vi "S7NetCom Simple Test Harness.vi"() -> ()   [LabVIEW 2014]
doc: "____\nCopyright (c) 2019 Hampel Software Engineering (HSE), released under BSD license. More info can be found on https://dokuwiki.hampel-soft.com/code/hse/s7netcom. Original code published by Marc Christenson, Sisu Devices."
uses:
  Controls/S7_Variable_Type.ctl
  Controls/S7_Memory_Area.ctl
  Controls/S7_Start_Address.ctl
  API/Write Data - Boolean (Scalar).vi
  API/Write Data - String.vi
  API/Write Data - DTL (Scalar).vi
  API/Write Data - Siemens Date & Time (Scalar).vi
  API/Write Data - Byte (Scalar).vi
  API/Write Data - Word (Scalar).vi
  API/Write Data - Real (Scalar).vi
  API/Write Data - Real (1D Array).vi
  API/Read Data - Boolean (Scalar).vi
  API/Read Data - String.vi
  API/Read Data - DTL (Scalar).vi
  API/Read Data - Siemens Date&Time (Scalar).vi
  API/Read Data - Byte (Scalar).vi
  API/Read Data - Word (Scalar).vi
  API/Read Data - Real (Scalar).vi
  API/Read Data - Real (1D Array).vi
  S7NetCom.lvclass
panel:
  in  "Cont TO":i32=250
  in  "Count":u16=1 caption="Read Length"
  out "Seq No":u16
  in  "RAW Var Type":T1=enum."BYTE"
  in  "Memory Area":T2=132 items=["P Area"=128, "I Area"=129, "O Area"=130, "M Area"=131, "DB Area"=132, "Counter"=40, "Timer"=41]
  in  "Start Address":T3
  in  "Data Block #":u16=1
  in  "Bit Offset":u8
  in  "Cont Variable Type":T1=enum."BYTE" caption="Variable Type"
  in  "Cont Memory Area":T2=132 caption="Memory Area" items=["P Area"=128, "I Area"=129, "O Area"=130, "M Area"=131, "DB Area"=132, "Counter"=40, "Timer"=41]
  in  "Cont Start Address":T3 caption="Start Address"
  in  "Cont Read Length":u16=1 caption="Read Length"
  in  "Cont Data Block #":u16=1 caption="Data Block #"
  in  "Cont Bit Offset":u8 caption="Bit Offset"
  in  "Tab Control TX":T4(tab)
  in  "TX Data":u32[](array[numeric])
  in  "Btn_WriteRaw":bool
  in  "Btn_WriteBOOL":bool
  in  "Boolean Value (TX)":bool
  out "Boolean Value (RX)":bool
  in  "Btn_ReadBOOL":bool
  in  "Btn_WriteBYTE":bool
  in  "Byte Value (TX)":u8
  out "Byte Value (RX)":u8
  in  "Btn_ReadBYTE":bool
  in  "Btn_WriteWORD":bool
  in  "Word Value (TX)":u16
  out "Word Value (RX)":u16
  in  "Btn_ReadWORD":bool
  in  "Btn_WriteREAL":bool
  in  "Real Value (TX)":sgl
  out "Real Value (RX)":sgl
  in  "Btn_ReadREAL":bool
  in  "Real Values (TX)":sgl[](array[numeric])
  in  "Btn_WriteREALArray":bool
  in  "Btn_ReadREALArray":bool
  out "Real Values (RX)":sgl[](array[numeric])
  in  "String Read Length":u16
  out "String Value (RX)":string
  in  "String Value (TX)":string
  in  "Btn_WriteSTRING":bool
  in  "Btn_ReadSTRING":bool
  in  "Btn_ReadDTL":bool
  out "DTL Value (RX)":timestamp
  in  "DTL (TX)":timestamp
  in  "Btn_Write DTL":bool
  in  "Date & Time (TX)":timestamp
  in  "Btn_Write D&T":bool
  in  "Btn_ReadD&T":bool
  out "Date&Time Value (RX)":timestamp
  out "Read/Write Error out":errorcluster
  out "Real (32bit)":sgl
  in  "Rack":u8
  out "Bits (1st byte)":bool[](array[boolean])
  out "Char's":string[](array[string])
  out "String":string
  in  "stop":bool
  out "U32":i32[](array[numeric]) format="%.0x"
  out "Error out":errorcluster caption="Read Continuously Error out"
  in  "IP Address":string
  in  "Port":i32=102
  in  "Slot":u8
  in  "Timeout":i32=5000
  # "Connection"
  # "Read Continuously"
  # "Read / Write"
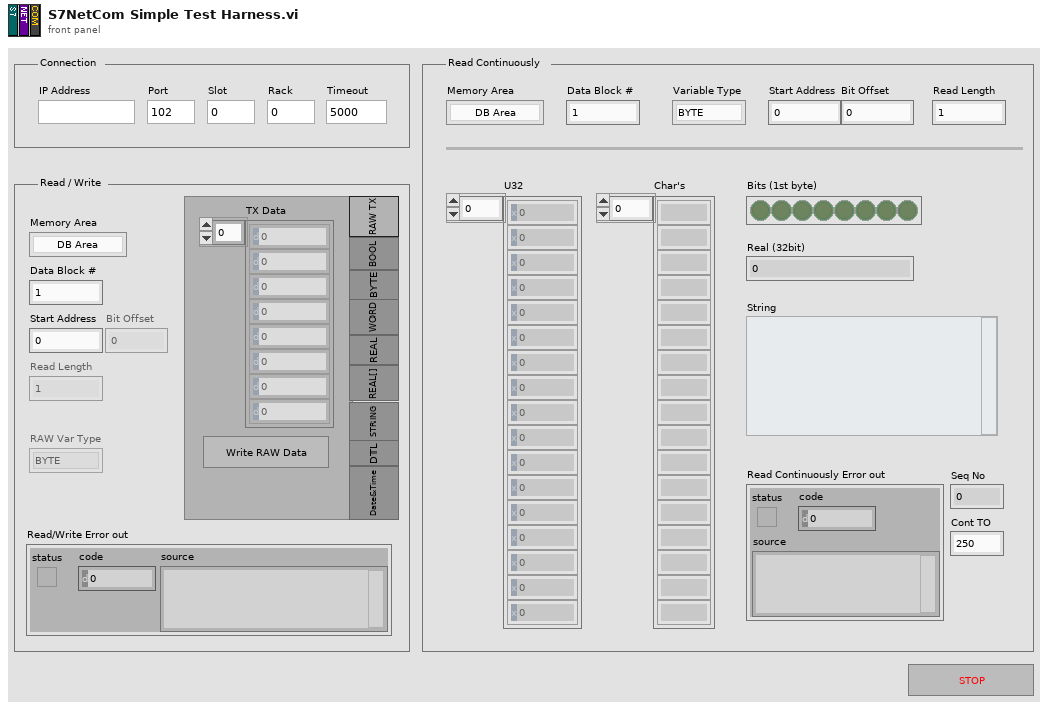
[diagram p1: front panel]
types:
  T1 = typedef "S7NetCom.lvclass/S7_Variable_Type.ctl" = enum8{"---", "BIT", "BYTE", "CHAR", "WORD", "INT", "DWORD", "DINT", "REAL"}
  T2 = typedef "S7NetCom.lvclass/S7_Memory_Area.ctl" = u8
  T3 = typedef "S7NetCom.lvclass/S7_Start_Address.ctl" = u16
  T4 = enum32{"RAW TX", "BOOL", "BYTE", "WORD", "REAL", "REAL[]", "STRING", "DTL", "Date&Time"}
  T5 = enum8{"Enabled", "Disabled", "Disabled and Grayed Out"}
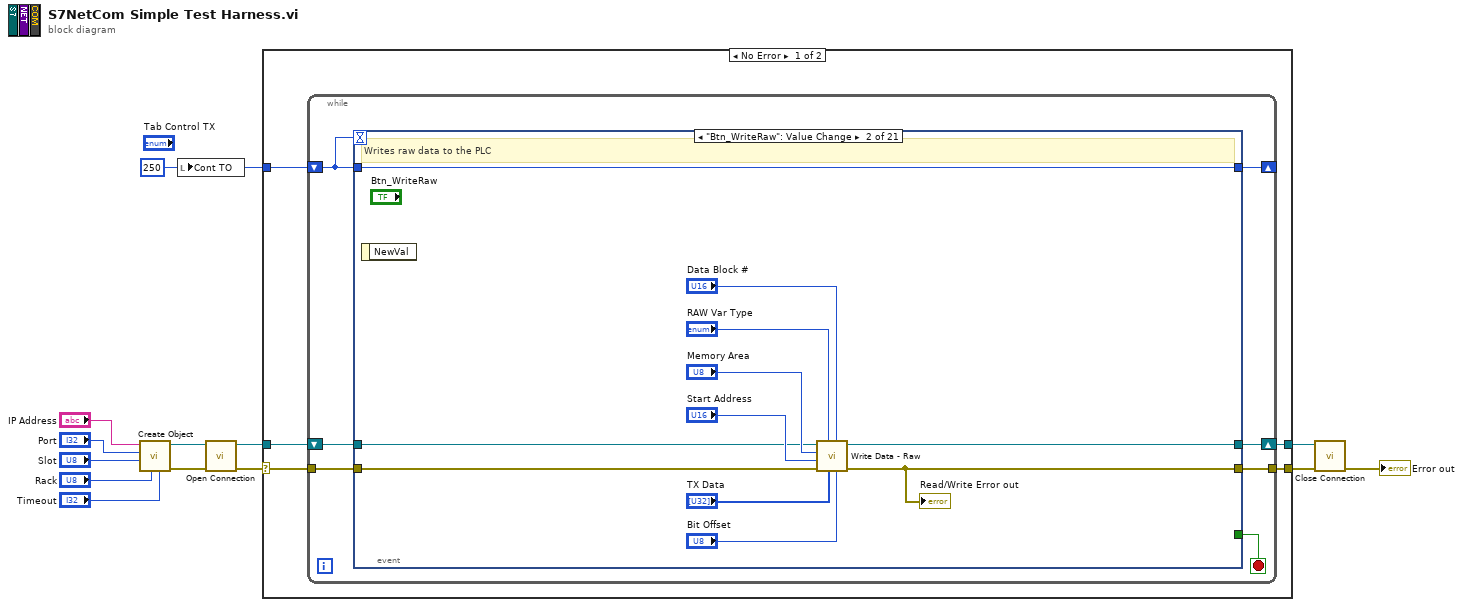
[diagram p0: block diagram]
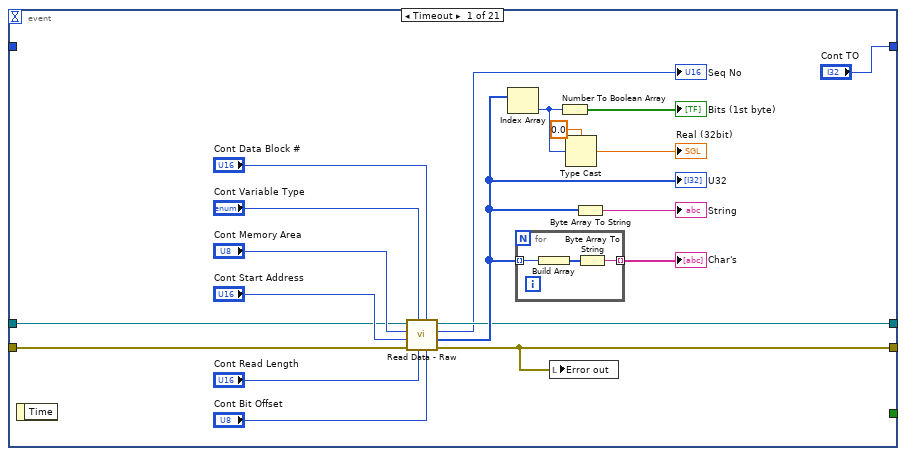
[diagram p2: hidden frame]
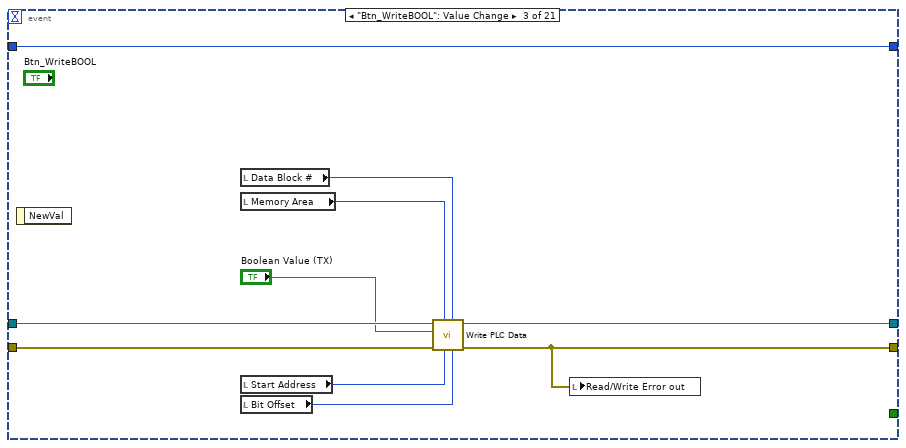
[diagram p3: hidden frame]
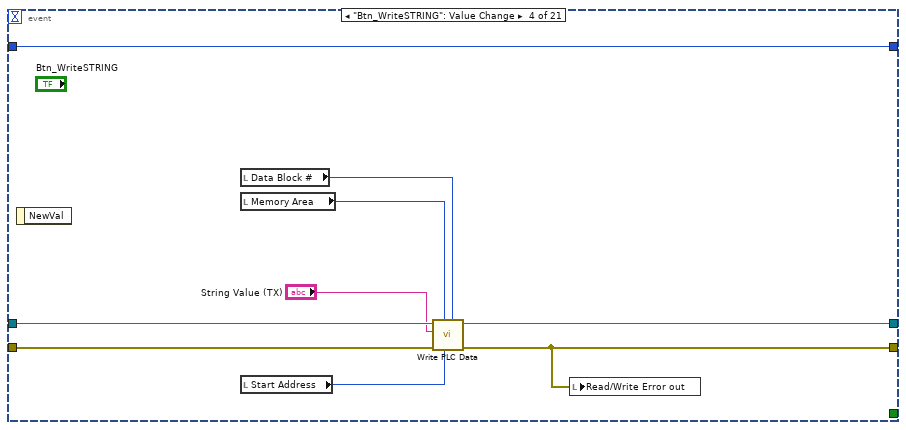
[diagram p4: hidden frame]
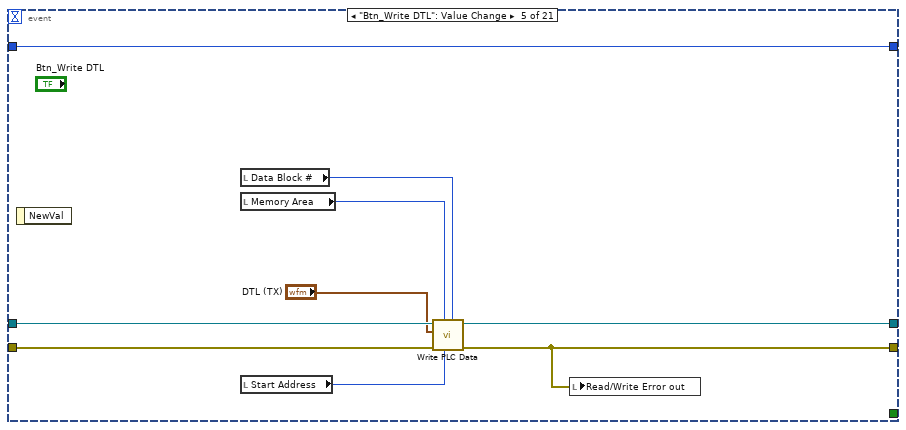
[diagram p5: hidden frame]
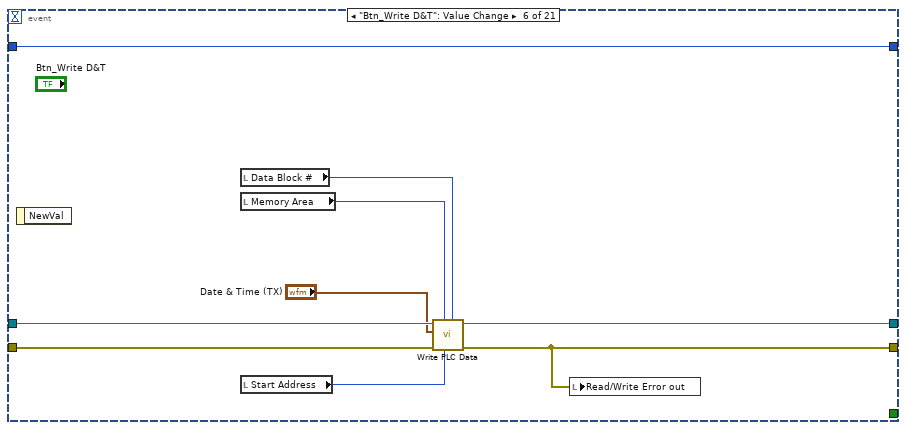
[diagram p6: hidden frame]
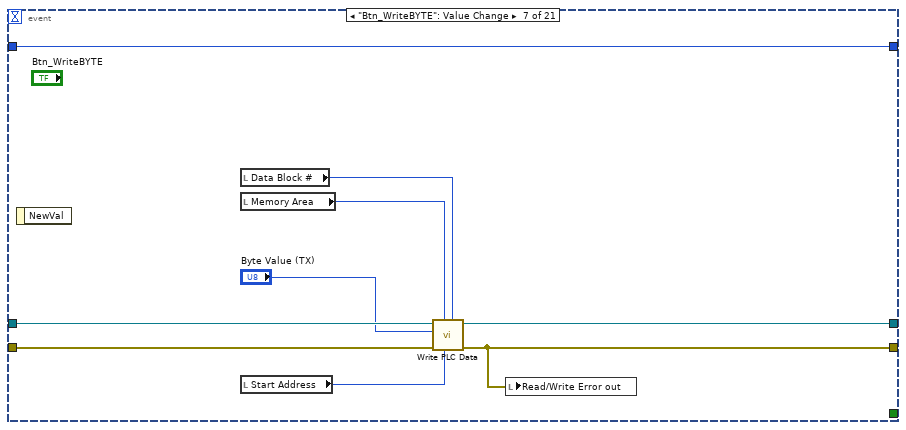
[diagram p7: hidden frame]
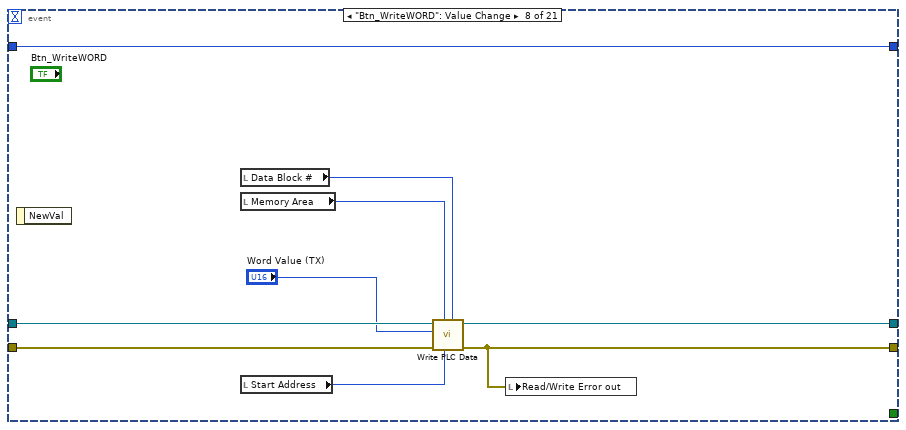
[diagram p8: hidden frame]
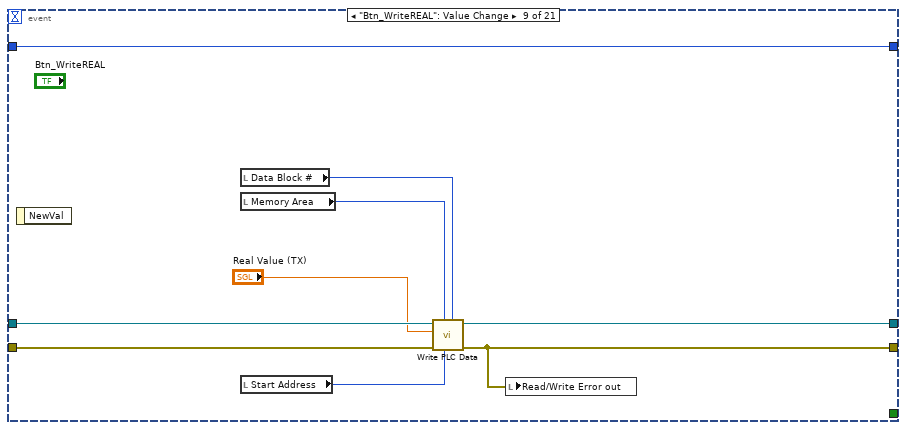
[diagram p9: hidden frame]
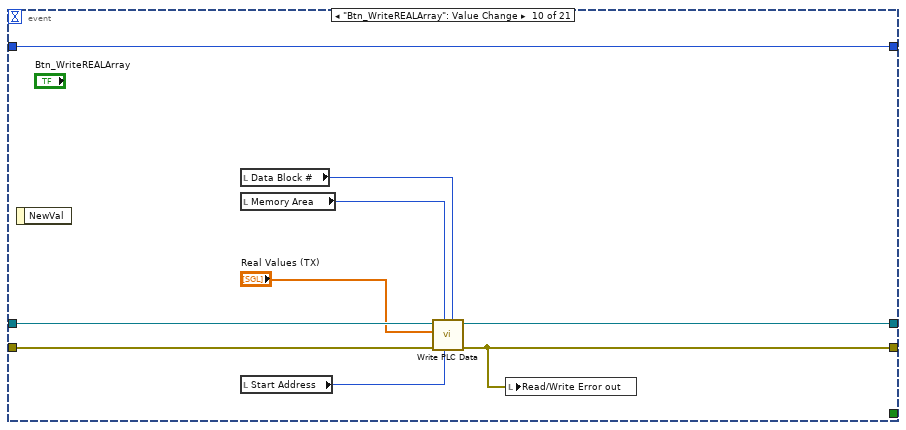
[diagram p10: hidden frame]
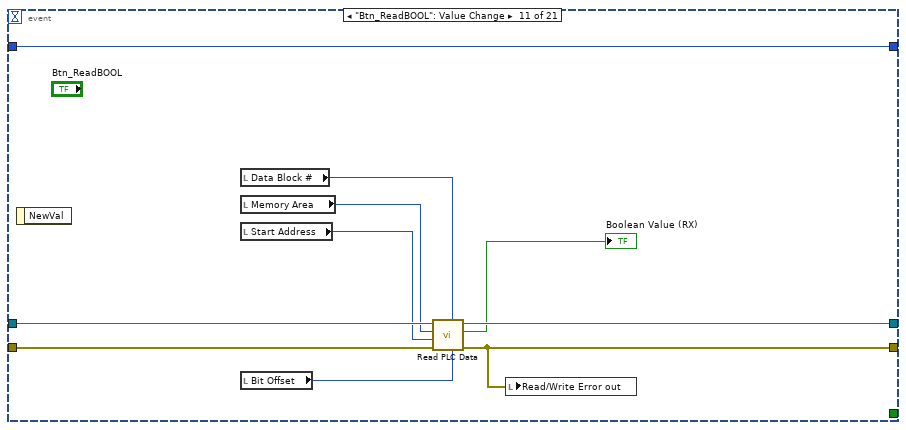
[diagram p11: hidden frame]
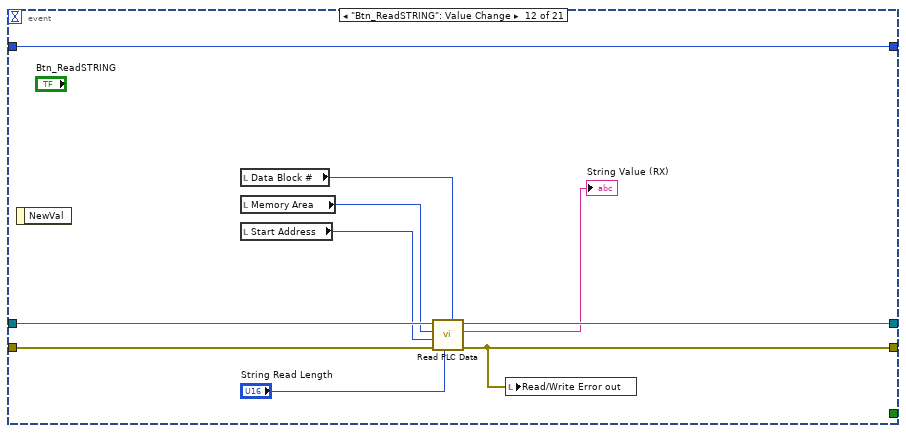
[diagram p12: hidden frame]
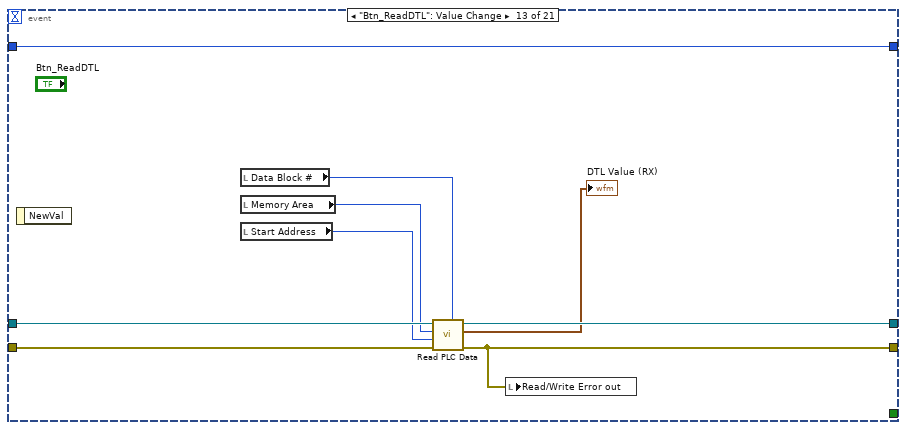
[diagram p13: hidden frame]
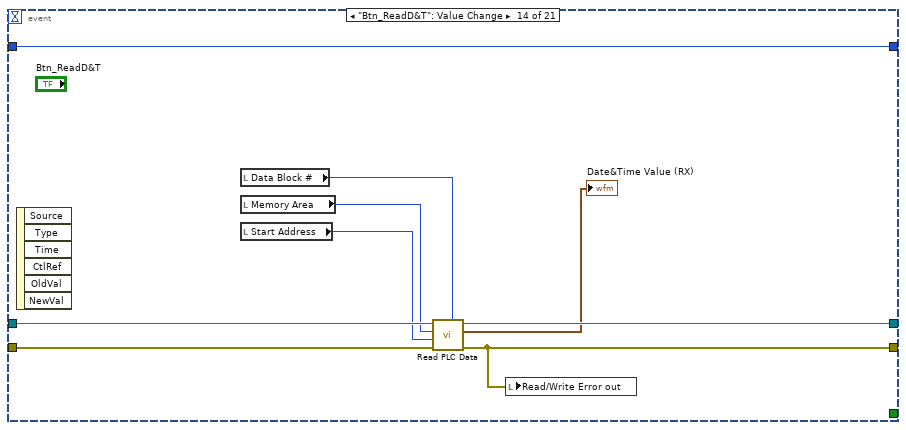
[diagram p14: hidden frame]
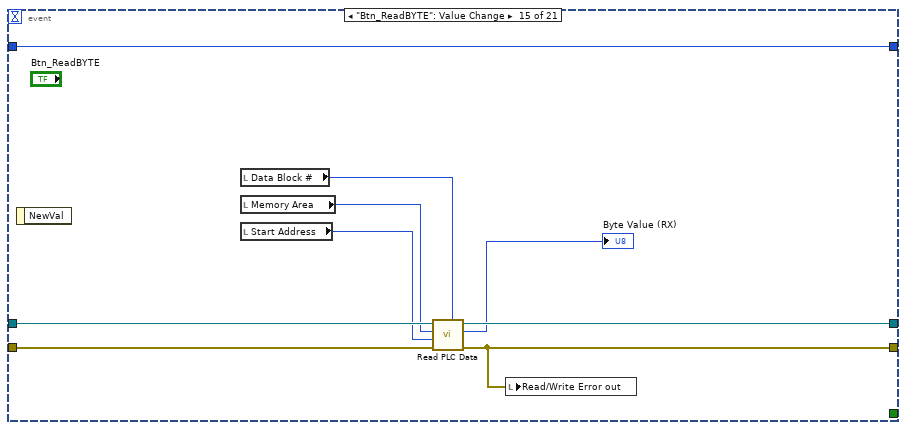
[diagram p15: hidden frame]
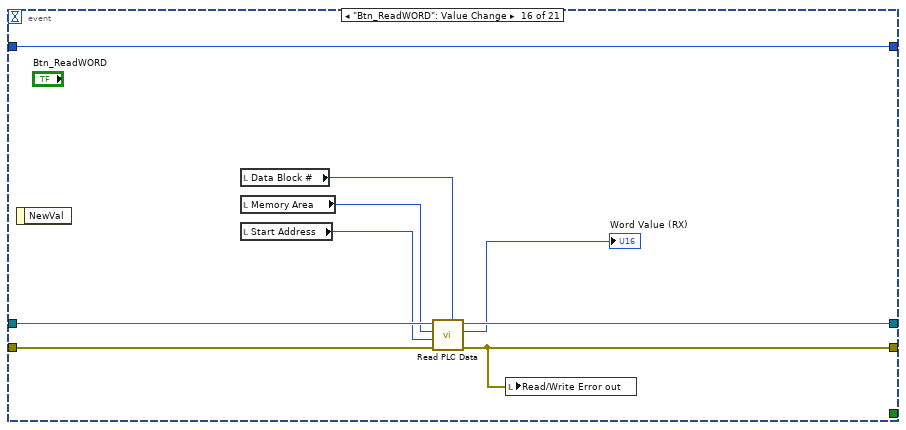
[diagram p16: hidden frame]
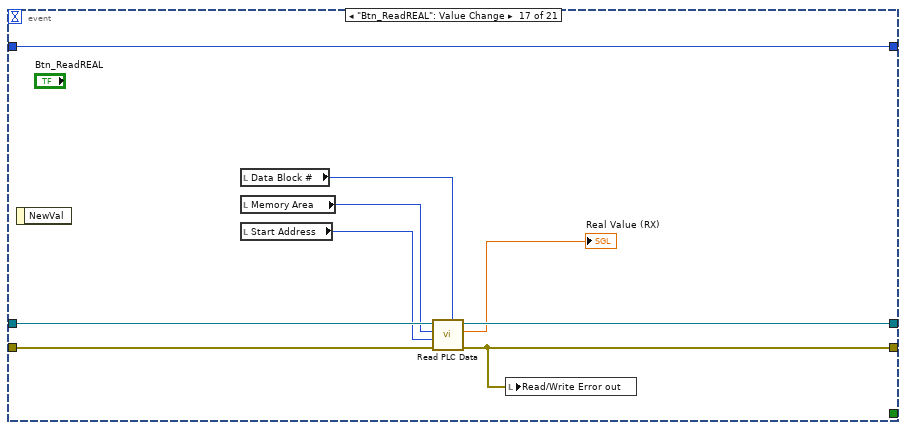
[diagram p17: hidden frame]
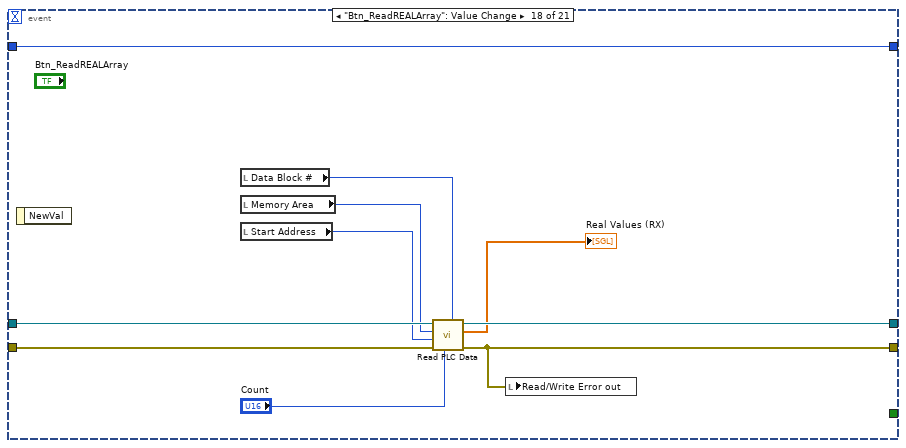
[diagram p18: hidden frame]
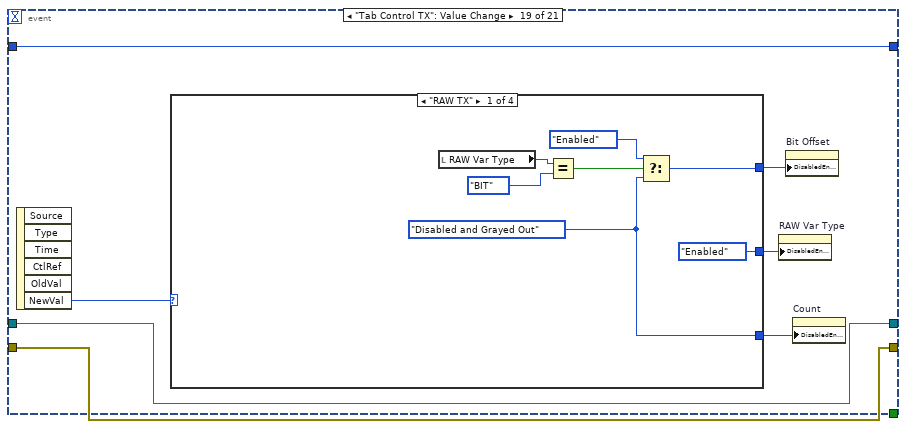
[diagram p19: hidden frame]
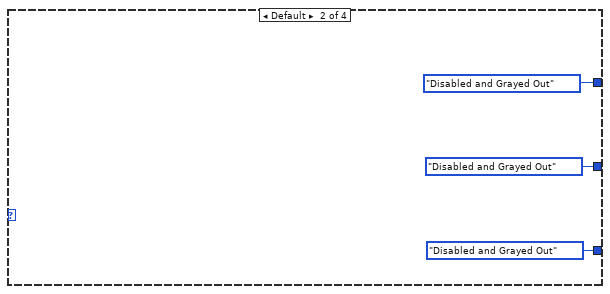
[diagram p20: hidden frame]
diagram:
  w1 = 250
  n1 = call "Create Object.vi"("Timeout"="Timeout", "Rack"="Rack", "Slot"="Slot", "Port"="Port", "IP Address"="IP Address") -> ("error out"=w10:errorcluster, "S7NetCom out"=w13:refnum<class "S7NetCom.lvclass">)  [unwired: 5 in]
  n2 = local write "Cont TO"(w1) -> ()
  n3 = call "Open Connection.vi"("error in"=w10, "S7NetCom in"=w13) -> ("error out"=w9:errorcluster, "S7NetCom out"=w12:refnum<class "S7NetCom.lvclass">)  [unwired: 8 in]
  n4 = case shown="No Error" w9 {
    selector: w9 -> [w15 w240]
    tunnel: w12 -> [w18 w241]
    tunnel: [w17 w241] -> w11
    tunnel: [w16 w240] -> w8
    tunnel: w1 -> [w14 _]
    frame No Error {
      n5 = while {
        shift-right: [w23] -> w17
        shift-left: w18 -> [w25]
        tunnel: [w21] -> w16
        tunnel: w15 -> [w22]
        shift-right: [w19] -> _
        shift-left: w14 -> [w20]
        stop <- w24 stop-if-true
        n6 = event shown="[1] \"Btn_WriteRaw\": Value Change" {
          selector: _ -> [_ _ _ _ _ _ _ _ _ _ _ _ _ _ _ _ _ _ _ _ _]
          dyn-events: _ -> [_ _ _ _ _ _ _ _ _ _ _ _ _ _ _ _ _ _ _ _ _]
          timeout: w20 -> [_ _ _ _ _ _ _ _ _ _ _ _ _ _ _ _ _ _ _ _ _]
          tunnel: w25 -> [w32 w51 w67 w76 w85 w94 w103 w112 w121 w130 w140 w150 w159 w168 w177 w186 w195 w205 w207 w231 w238]
          tunnel: [_ _ _ _ _ _ _ _ _ _ _ _ _ _ _ _ _ _ _ _ w239] -> w24
          tunnel: [w31 w50 w65 w74 w83 w92 w101 w110 w119 w128 w138 w148 w157 w166 w175 w184 w193 w203 w207 w231 w238] -> w23
          tunnel: w22 -> [w29 w52 w68 w77 w86 w95 w104 w113 w122 w131 w141 w151 w160 w169 w178 w187 w196 w206 w208 w232 w237]
          tunnel: [w30 w49 w66 w75 w84 w93 w102 w111 w120 w129 w139 w149 w158 w167 w176 w185 w194 w204 w208 w232 w237] -> w21
          tunnel: w20 -> [_ w48 w59 w70 w79 w88 w96 w105 w114 w123 w132 w144 w153 w162 w170 w179 w188 w197 w213 w233 w236]
          tunnel: ["Cont TO" w48 w59 w70 w79 w88 w96 w105 w114 w123 w132 w144 w153 w162 w170 w179 w188 w197 w213 w233 w236] -> w19
          event Timeout {
            n7 = event-data() -> ()  [unwired: 1 in, 1 out]
            n8 = call "Read Data - Raw.vi"("Bit Offset"="Cont Bit Offset", "Data Block #"="Cont Data Block #", "Read Length"="Cont Read Length", "Variable Type"="Cont Variable Type", "error in (no error)"=w29, "Start Address"="Cont Start Address", "Memory Area"="Cont Memory Area", "S7 in"=w32) -> ("error out"=w30:errorcluster, "Read Data"=w36:i32[], "Sequence No"=→"Seq No":u16, "S7 out"=w31:refnum<class "S7NetCom.lvclass">)
            "U32" <- w36
            n9 = Index Array(array=w36) -> (element=w35:i32)  [unwired: 1 in]
            n10 = for {
              tunnel: w36 -> [w47] mode=indexing
              tunnel: [w46] -> w43 mode=indexing
              n11 = Build Array(w47) -> (w45:i32[])
              n12 = Byte Array To String(unsigned byte array=w45) -> (string=w46:string)
            }
            "Char's" <- w43
            n13 = local write "Error out"(w30) -> ()
            n14 = Number To Boolean Array(number=w35) -> (Boolean array=→"Bits (1st byte)":bool[])
            n15 = Type Cast(type=sgl 0.0 ("Real (32bit)"), x=w35) -> (*(type *) &x=→"Real (32bit)":sgl)
            n16 = Byte Array To String(unsigned byte array=w36) -> (string=→"String":string)
          }
          event "Btn_WriteRaw": Value Change {
            # "Writes raw data to the PLC"
            n17 = event-data() -> ()  [unwired: 1 in, 1 out]
            n18 = call "Write Data - Raw.vi"("Bit Offset"="Bit Offset", "Data Block #"="Data Block #", "Write Data"="TX Data", "Variable Type"="RAW Var Type", "error in (no error)"=w52, "Start Address"="Start Address", "Memory Area"="Memory Area", "S7 in"=w51) -> ("error out"=w49:errorcluster, "S7 out"=w50:refnum<class "S7NetCom.lvclass">)  [unwired: 2 in]
            "Read/Write Error out" <- w49
          }
          event "Btn_WriteBOOL": Value Change {
            n19 = event-data() -> ()  [unwired: 1 in, 1 out]
            n20 = local read "Data Block #"() -> (w64:u16)
            n21 = local read "Memory Area"() -> (w61:T2)
            n22 = local read "Start Address"() -> (w62:T3)
            n23 = local read "Bit Offset"() -> (w63:u8)
            n24 = call-poly "Write PLC Data.vi"("Bit Offset"=w63, "Data Block #"=w64, "Start Address"=w62, "Memory Area"=w61, "error in (no error)"=w68, "Value"="Boolean Value (TX)", "S7 in"=w67) -> ("error out"=w66:errorcluster, "S7 out"=w65:refnum<class "S7NetCom.lvclass">)  [unwired: 3 in]
            n25 = local write "Read/Write Error out"(w66) -> ()
          }
          event "Btn_WriteSTRING": Value Change {
            n26 = event-data() -> ()  [unwired: 1 in, 1 out]
            n27 = local read "Data Block #"() -> (w73:u16)
            n28 = local read "Memory Area"() -> (w71:T2)
            n29 = local read "Start Address"() -> (w72:T3)
            n30 = call-poly "Write PLC Data.vi"("Data Block #"=w73, "Start Address"=w72, "Memory Area"=w71, "error in (no error)"=w77, "String"="String Value (TX)", "S7 in"=w76) -> ("error out"=w75:errorcluster, "S7 out"=w74:refnum<class "S7NetCom.lvclass">)  [unwired: 4 in]
            n31 = local write "Read/Write Error out"(w75) -> ()
          }
          event "Btn_Write DTL": Value Change {
            n32 = event-data() -> ()  [unwired: 1 in, 1 out]
            n33 = local read "Data Block #"() -> (w82:u16)
            n34 = local read "Memory Area"() -> (w80:T2)
            n35 = local read "Start Address"() -> (w81:T3)
            n36 = call-poly "Write PLC Data.vi"("Data Block #"=w82, "Start Address"=w81, "Memory Area"=w80, "error in (no error)"=w86, "Value"="DTL (TX)", "S7 in"=w85) -> ("error out"=w84:errorcluster, "S7 out"=w83:refnum<class "S7NetCom.lvclass">)  [unwired: 4 in]
            n37 = local write "Read/Write Error out"(w84) -> ()
          }
          event "Btn_Write D&T": Value Change {
            n38 = event-data() -> ()  [unwired: 1 in, 1 out]
            n39 = local read "Data Block #"() -> (w91:u16)
            n40 = local read "Memory Area"() -> (w89:T2)
            n41 = local read "Start Address"() -> (w90:T3)
            n42 = call-poly "Write PLC Data.vi"("Data Block #"=w91, "Start Address"=w90, "Memory Area"=w89, "error in (no error)"=w95, "Value"="Date & Time (TX)", "S7 in"=w94) -> ("error out"=w93:errorcluster, "S7 out"=w92:refnum<class "S7NetCom.lvclass">)  [unwired: 4 in]
            n43 = local write "Read/Write Error out"(w93) -> ()
          }
          event "Btn_WriteBYTE": Value Change {
            n44 = event-data() -> ()  [unwired: 1 in, 1 out]
            n45 = local read "Data Block #"() -> (w99:u16)
            n46 = local read "Memory Area"() -> (w100:T2)
            n47 = local read "Start Address"() -> (w98:T3)
            n48 = call-poly "Write PLC Data.vi"("Data Block #"=w99, "Start Address"=w98, "Memory Area"=w100, "error in (no error)"=w104, "Value"="Byte Value (TX)", "S7 in"=w103) -> ("error out"=w102:errorcluster, "S7 out"=w101:refnum<class "S7NetCom.lvclass">)  [unwired: 4 in]
            n49 = local write "Read/Write Error out"(w102) -> ()
          }
          event "Btn_WriteWORD": Value Change {
            n50 = event-data() -> ()  [unwired: 1 in, 1 out]
            n51 = local read "Data Block #"() -> (w108:u16)
            n52 = local read "Memory Area"() -> (w109:T2)
            n53 = local read "Start Address"() -> (w107:T3)
            n54 = call-poly "Write PLC Data.vi"("Data Block #"=w108, "Start Address"=w107, "Memory Area"=w109, "error in (no error)"=w113, "Value"="Word Value (TX)", "S7 in"=w112) -> ("error out"=w111:errorcluster, "S7 out"=w110:refnum<class "S7NetCom.lvclass">)  [unwired: 4 in]
            n55 = local write "Read/Write Error out"(w111) -> ()
          }
          event "Btn_WriteREAL": Value Change {
            n56 = event-data() -> ()  [unwired: 1 in, 1 out]
            n57 = local read "Data Block #"() -> (w117:u16)
            n58 = local read "Memory Area"() -> (w118:T2)
            n59 = local read "Start Address"() -> (w116:T3)
            n60 = call-poly "Write PLC Data.vi"("Data Block #"=w117, "Start Address"=w116, "Memory Area"=w118, "error in (no error)"=w122, "Value"="Real Value (TX)", "S7 in"=w121) -> ("error out"=w120:errorcluster, "S7 out"=w119:refnum<class "S7NetCom.lvclass">)  [unwired: 4 in]
            n61 = local write "Read/Write Error out"(w120) -> ()
          }
          event "Btn_WriteREALArray": Value Change {
            n62 = event-data() -> ()  [unwired: 1 in, 1 out]
            n63 = local read "Data Block #"() -> (w126:u16)
            n64 = local read "Memory Area"() -> (w127:T2)
            n65 = local read "Start Address"() -> (w125:T3)
            n66 = call-poly "Write PLC Data.vi"("Data Block #"=w126, "Start Address"=w125, "Memory Area"=w127, "error in (no error)"=w131, "Values"="Real Values (TX)", "S7 in"=w130) -> ("error out"=w129:errorcluster, "S7 out"=w128:refnum<class "S7NetCom.lvclass">)  [unwired: 4 in]
            n67 = local write "Read/Write Error out"(w129) -> ()
          }
          event "Btn_ReadBOOL": Value Change {
            n68 = event-data() -> ()  [unwired: 1 in, 1 out]
            n69 = local read "Data Block #"() -> (w136:u16)
            n70 = local read "Memory Area"() -> (w137:T2)
            n71 = local read "Start Address"() -> (w135:T3)
            n72 = local read "Bit Offset"() -> (w133:u8)
            n73 = call-poly "Read PLC Data.vi"("Bit Offset"=w133, "Data Block #"=w136, "error in (no error)"=w141, "Start Address"=w135, "Memory Area"=w137, "S7 in"=w140) -> ("error out"=w139:errorcluster, "Boolean Value"=→"Boolean Value (RX)":bool, "S7 out"=w138:refnum<class "S7NetCom.lvclass">)  [unwired: 3 in]
            n74 = local write "Read/Write Error out"(w139) -> ()
          }
          event "Btn_ReadSTRING": Value Change {
            n75 = event-data() -> ()  [unwired: 1 in, 1 out]
            n76 = local read "Data Block #"() -> (w146:u16)
            n77 = local read "Memory Area"() -> (w147:T2)
            n78 = local read "Start Address"() -> (w145:T3)
            n79 = call-poly "Read PLC Data.vi"("Data Block #"=w146, "Read Length"="String Read Length", "error in (no error)"=w151, "Start Address"=w145, "Memory Area"=w147, "S7 in"=w150) -> ("error out"=w149:errorcluster, "String Value"=→"String Value (RX)":string, "S7 out"=w148:refnum<class "S7NetCom.lvclass">)  [unwired: 3 in]
            n80 = local write "Read/Write Error out"(w149) -> ()
          }
          event "Btn_ReadDTL": Value Change {
            n81 = event-data() -> ()  [unwired: 1 in, 1 out]
            n82 = local read "Data Block #"() -> (w155:u16)
            n83 = local read "Memory Area"() -> (w156:T2)
            n84 = local read "Start Address"() -> (w154:T3)
            n85 = call-poly "Read PLC Data.vi"("Data Block #"=w155, "error in (no error)"=w160, "Start Address"=w154, "Memory Area"=w156, "S7 in"=w159) -> ("error out"=w158:errorcluster, "Time Stamp"=→"DTL Value (RX)":timestamp, "S7 out"=w157:refnum<class "S7NetCom.lvclass">)  [unwired: 4 in]
            n86 = local write "Read/Write Error out"(w158) -> ()
          }
          event "Btn_ReadD&T": Value Change {
            n87 = event-data() -> ()  [unwired: 1 in, 6 out]
            n88 = local read "Data Block #"() -> (w164:u16)
            n89 = local read "Memory Area"() -> (w165:T2)
            n90 = local read "Start Address"() -> (w163:T3)
            n91 = call-poly "Read PLC Data.vi"("Data Block #"=w164, "error in (no error)"=w169, "Start Address"=w163, "Memory Area"=w165, "S7 in"=w168) -> ("error out"=w167:errorcluster, "Time Stamp"=→"Date&Time Value (RX)":timestamp, "S7 out"=w166:refnum<class "S7NetCom.lvclass">)  [unwired: 4 in]
            n92 = local write "Read/Write Error out"(w167) -> ()
          }
          event "Btn_ReadBYTE": Value Change {
            n93 = event-data() -> ()  [unwired: 1 in, 1 out]
            n94 = local read "Data Block #"() -> (w173:u16)
            n95 = local read "Memory Area"() -> (w174:T2)
            n96 = local read "Start Address"() -> (w172:T3)
            n97 = call-poly "Read PLC Data.vi"("Data Block #"=w173, "error in (no error)"=w178, "Start Address"=w172, "Memory Area"=w174, "S7 in"=w177) -> ("error out"=w176:errorcluster, "Byte Value"=→"Byte Value (RX)":u8, "S7 out"=w175:refnum<class "S7NetCom.lvclass">)  [unwired: 4 in]
            n98 = local write "Read/Write Error out"(w176) -> ()
          }
          event "Btn_ReadWORD": Value Change {
            n99 = event-data() -> ()  [unwired: 1 in, 1 out]
            n100 = local read "Data Block #"() -> (w182:u16)
            n101 = local read "Memory Area"() -> (w183:T2)
            n102 = local read "Start Address"() -> (w181:T3)
            n103 = call-poly "Read PLC Data.vi"("Data Block #"=w182, "error in (no error)"=w187, "Start Address"=w181, "Memory Area"=w183, "S7 in"=w186) -> ("error out"=w185:errorcluster, "Word Value"=→"Word Value (RX)":u16, "S7 out"=w184:refnum<class "S7NetCom.lvclass">)  [unwired: 4 in]
            n104 = local write "Read/Write Error out"(w185) -> ()
          }
          event "Btn_ReadREAL": Value Change {
            n105 = event-data() -> ()  [unwired: 1 in, 1 out]
            n106 = local read "Data Block #"() -> (w191:u16)
            n107 = local read "Memory Area"() -> (w192:T2)
            n108 = local read "Start Address"() -> (w190:T3)
            n109 = call-poly "Read PLC Data.vi"("Data Block #"=w191, "error in (no error)"=w196, "Start Address"=w190, "Memory Area"=w192, "S7 in"=w195) -> ("error out"=w194:errorcluster, "Real Value"=→"Real Value (RX)":sgl, "S7 out"=w193:refnum<class "S7NetCom.lvclass">)  [unwired: 4 in]
            n110 = local write "Read/Write Error out"(w194) -> ()
          }
          event "Btn_ReadREALArray": Value Change {
            n111 = event-data() -> ()  [unwired: 1 in, 1 out]
            n112 = local read "Data Block #"() -> (w201:u16)
            n113 = local read "Memory Area"() -> (w202:T2)
            n114 = local read "Start Address"() -> (w199:T3)
            n115 = call-poly "Read PLC Data.vi"("Data Block #"=w201, "Count"="Count", "error in (no error)"=w206, "Start Address"=w199, "Memory Area"=w202, "S7 in"=w205) -> ("error out"=w204:errorcluster, "Real Values"=→"Real Values (RX)":sgl[], "S7 out"=w203:refnum<class "S7NetCom.lvclass">)  [unwired: 3 in]
            n116 = local write "Read/Write Error out"(w204) -> ()
          }
          event "Tab Control TX": Value Change {
            n117 = event-data() -> ("NewVal"=w212:T4)  [unwired: 1 in, 5 out]
            n118 = case shown="\"RAW TX\"" w212 {
              tunnel: [w216 T5."Disabled and Grayed Out" ("Disabled") T5."Disabled and Grayed Out" ("Disabled") T5."Enabled" ("Disabled")] -> w211
              tunnel: [T5."Enabled" ("Disabled") T5."Disabled and Grayed Out" ("Disabled") T5."Disabled and Grayed Out" ("Disabled") w227] -> w210
              tunnel: [w214 T5."Disabled and Grayed Out" ("Disabled") T5."Enabled" ("Disabled") w227] -> w209
              frame "RAW TX" {
                w214 = T5."Disabled and Grayed Out" ("Disabled")
                n119 = local read "RAW Var Type"() -> (w220:T1)
                n120 = Equal?(x=w220, y=S7_Variable_Type."BIT") -> (x = y?=w218:bool)
                n121 = Select(t=T5."Enabled" ("Disabled"), s=w218, f=w214) -> (s? t:f=w216:T5)
              }
              frame Default {
              }
              frame "REAL[]" {
              }
              frame "BOOL" {
                w227 = T5."Disabled and Grayed Out" ("Disabled")
              }
            }
            n122 = property on="RAW Var Type" class="Enum (strict)"("DisabledEnum"=w210) -> ()  [unwired: 2 in, 2 out]
            n123 = property on="Bit Offset" class="DigNum (strict)"("DisabledEnum"=w211) -> ()  [unwired: 2 in, 2 out]
            n124 = property on="Count" class="DigNum (strict)"("DisabledEnum"=w209) -> ()  [unwired: 2 in, 2 out]
          }
          event Value Change {
            n125 = event-data() -> ("NewVal"=w230:T1)  [unwired: 1 in, 5 out]
            n126 = case shown="\"---\", Default" w230 {
              tunnel: [T5."Disabled and Grayed Out" ("Disabled") T5."Enabled" ("Disabled")] -> w229
              frame "---", Default {
              }
              frame "BIT" {
              }
            }
            n127 = property on="Bit Offset" class="DigNum (strict)"("DisabledEnum"=w229) -> ()  [unwired: 2 in, 2 out]
          }
          event "stop": Value Change {
            n128 = event-data() -> ("NewVal"=w239:bool)  [unwired: 1 in]
          }
        }
      }
    }
    frame Error {
    }
  }
  n129 = call "Close Connection.vi"("error in (no error)"=w8, "S7NetCom in"=w11) -> ("error out"=→"Error out":errorcluster)  [unwired: 8 in, 1 out]
